vi "DIALOG BOX HFRR ADV.vi"(1 "Status":string="Warning:\nTrained and authorized users only! \nEnsure all positioners are tightened and specimens are mounted securely.\nMoving machinery can cause serious injuries - keep away when equipment is in operation. \n", 3 "error in":errorcluster) -> (8 "Continue":bool, 9 "Cancel":bool, 10 "error out":errorcluster)   [LabVIEW 2025]
panel:
  in  "Cancel":bool
  in  "Boolean":bool
  in  "Continue":bool
  # "Service Mode"
  # "CAUTION - Improper use of Service Mode could result in loss of Machine Operation , permanent Machine damage , or serious personal Injury."
  # "Service Mode is intended for qualified professionals to conduct diagnostics , repairs, \nand maintenance on HFRR ADV in a controlled and safe workshop environment.\n\nWhen working on a machine or using Service Mode always refer to the Manual for safety \nprecautions and procedures , and always adhere to industry best practices.\n\nVisit www.paltro.com/contact-forms/contact-customer-support for more information"
  # "Warning:\nTrained and authorized users only! Ensure all positioners are tightened and specimens are mounted securely.\nMoving machinery can cause serious injuries - keep away when equipment is in operation."
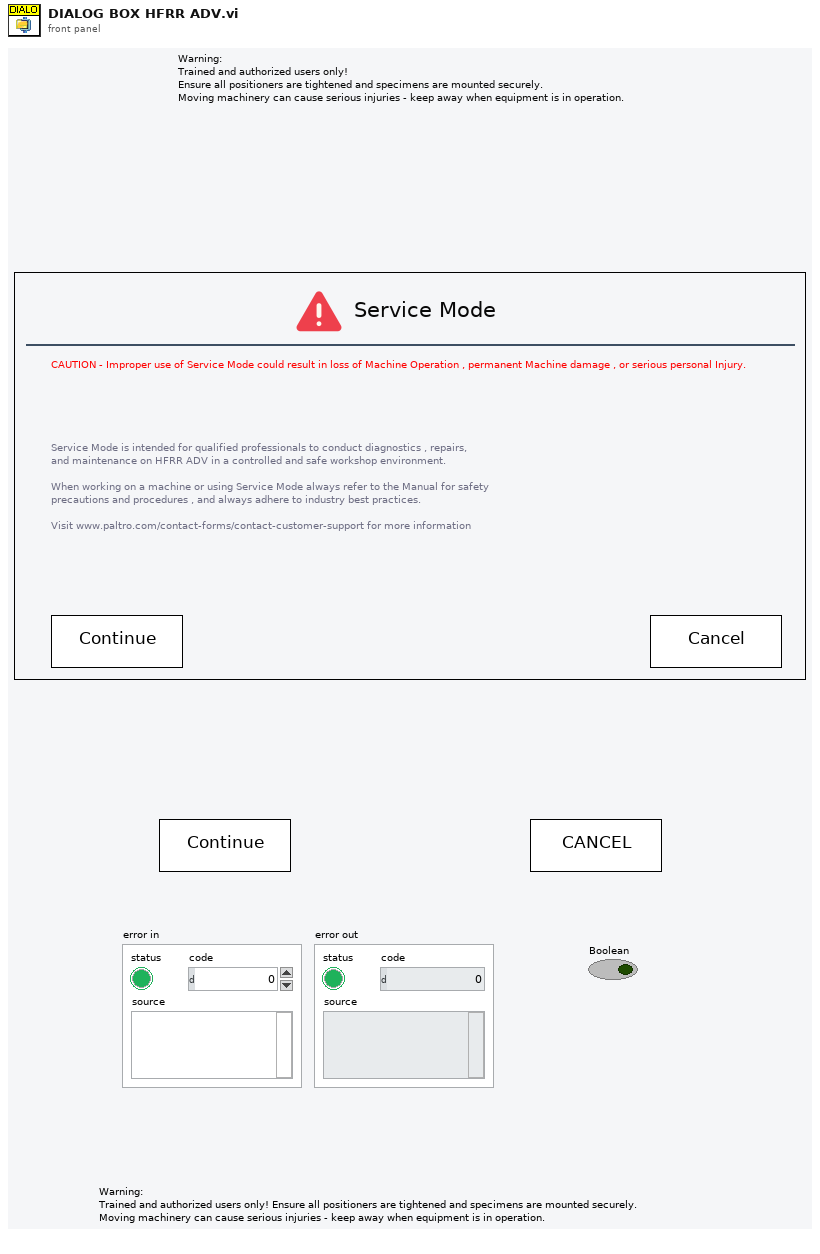
[diagram p1: front panel]
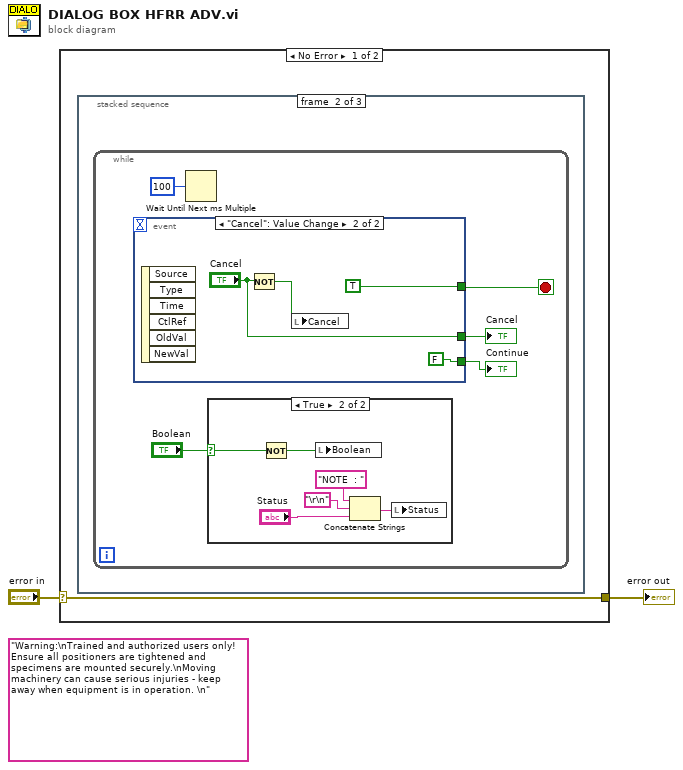
[diagram p0: block diagram]
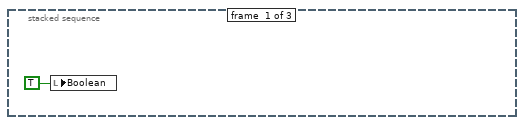
[diagram p2: hidden frame]
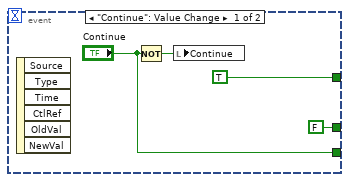
[diagram p4: hidden frame]
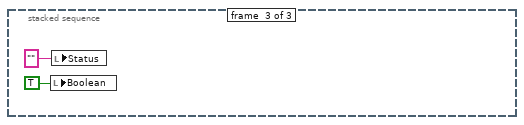
[diagram p5: hidden frame]
diagram:
  (unwired) "Warning:\nTrained and authorized users only! Ensure all positioners are tightened and specimens are mounted securely.\nMoving machinery can cause serious injuries - keep away when equipment is in operation. \n" ("message")
  n1 = case shown="No Error" "error in" {
    selector: "error in" -> [w3 _]
    tunnel: [w3 _] -> w1
    frame No Error {
      n2 = stacked-sequence {
        frame #0 {
          n3 = local write "Boolean"(TRUE ("Boolean")) -> ()
        }
        frame #1 {
          n4 = while {
            stop <- w8 stop-if-true
            n5 = event shown="[1] \"Cancel\": Value Change" {
              selector: _ -> [_ _]
              dyn-events: _ -> [_ _]
              timeout: _ -> [_ _]
              tunnel: [TRUE TRUE] -> w8
              tunnel: [FALSE ("Skip") "Cancel"] -> w6
              tunnel: ["Continue" FALSE] -> w5
              event "Continue": Value Change {
                n6 = event-data() -> ()  [unwired: 1 in, 6 out]
                n7 = Not(x="Continue") -> (.not. x?=w18:bool)
                n8 = local write "Continue"(w18) -> ()
              }
              event "Cancel": Value Change {
                n9 = event-data() -> ()  [unwired: 1 in, 6 out]
                n10 = Not(x="Cancel") -> (.not. x?=w22:bool)
                n11 = local write "Cancel"(w22) -> ()
              }
            }
            "Cancel" <- w6
            "Continue" <- w5
            n12 = Wait Until Next ms Multiple(millisecond multiple=100) -> ()  [unwired: 1 out]
            n13 = case shown="True" "Boolean" {
              selector: "Boolean" -> [_ w14]
              frame False {
              }
              frame True {
                n14 = Not(x=w14) -> (.not. x?=w13:bool)
                n15 = local write "Boolean"(w13) -> ()
                n16 = Concatenate Strings("NOTE  : ", "\r\n", "Status") -> (w12:string)
                n17 = local write "Status"(w12) -> ()
              }
            }
          }
        }
        frame #2 {
          n18 = local write "Boolean"(TRUE ("Boolean")) -> ()
          n19 = local write "Status"("") -> ()
        }
      }
    }
    frame Error {
    }
  }
  "error out" <- w1
